vi "Generation word specific.vi"(11 "Template Path":path) -> ()   [LabVIEW 2020]
uses:
  <vilib>/Utility/NIReport.llb/Report Type.ctl
  <vilib>/addons/_office/_exclsub.llb/font.ctl
  <vilib>/Utility/NIReport.llb/Append Text Table to Report (wrap).vi
  <vilib>/addons/_office/word.llb/Word Edit Cell ([str]).vi
  <vilib>/Utility/NIReport.llb/NI_report.lvclass
  <vilib>/Utility/NIReport.llb/NI_ReportGenerationCore.lvlib
  <vilib>/Utility/NIReport.llb/Word/NI_Word.lvclass
  <vilib>/addons/_office/NI_ReportGenerationToolkit.lvlib
panel:
  in  "Data Set Name":string
  in  "error in (no error)":errorcluster
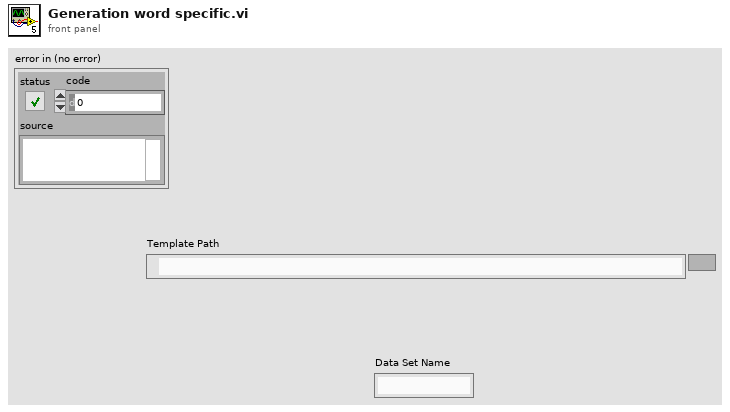
[diagram p1: front panel]
types:
  T1 = typedef "NI_ReportGenerationToolkit.lvlib/font.ctl" = cluster{"font name":string, "font size":dbl, "bold":u16, "italic":u16, "underline":u16, "strike through":u16, "font color":u32}
  T2 = typedef "NI_ReportGenerationCore.lvlib/Report Type.ctl" = enum16{"HTML", "Word", "Excel"}
  T3 = enum16{"maximized", "minimized", "normal", "no change"}
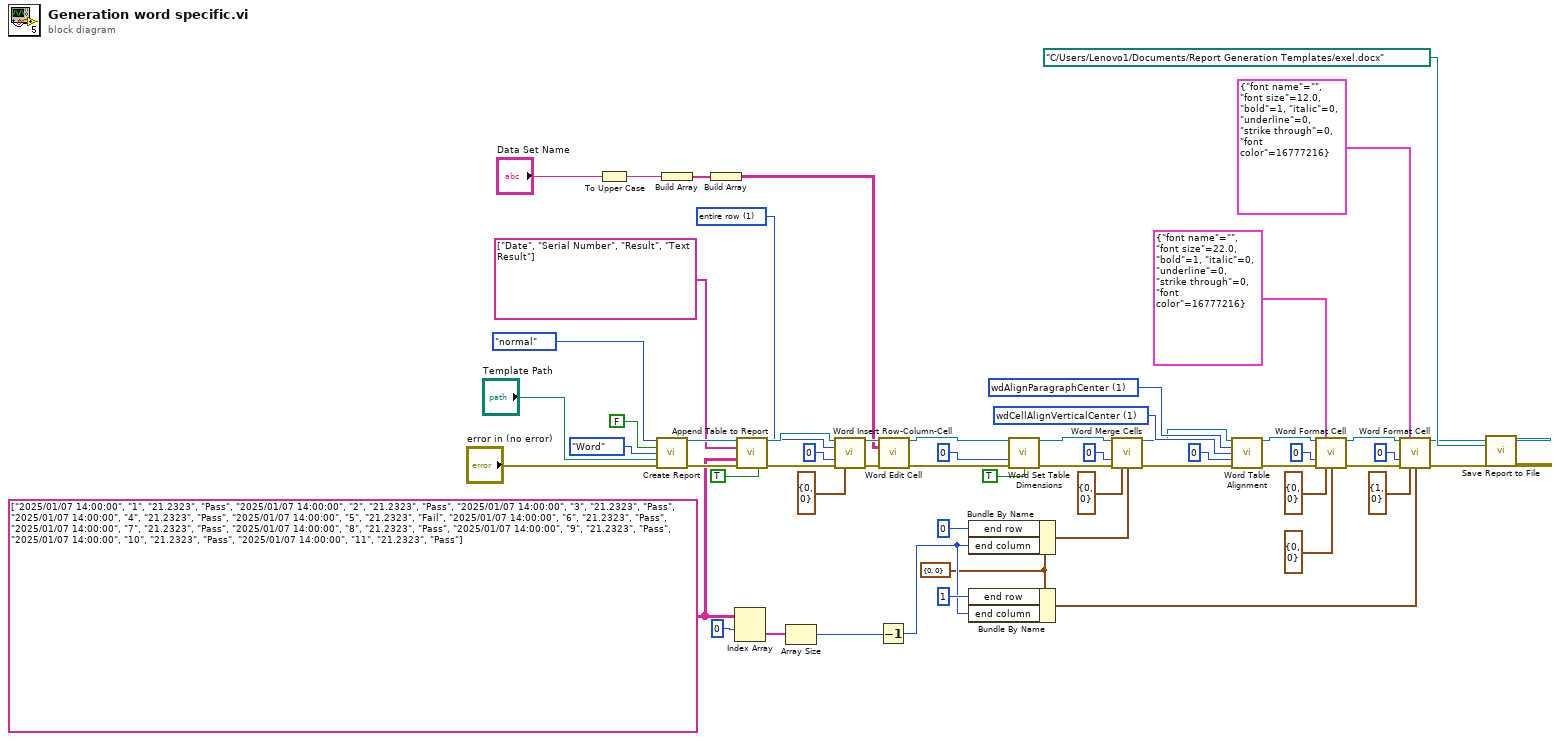
[diagram p0: block diagram]
diagram:
  w33 = u16 1 items=["shift cells right", "entire row", "entire column"] ("mode (entire column)")
  w1 = cluster{"end row":i32, "end column":i32} {"end row"=0, "end column"=0} ("end")
  w47 = 1 items=["wdCellAlignVerticalTop"=0, "wdCellAlignVerticalCenter"=1, "wdCellAlignVerticalBottom"=3] ("vertical alignment (top)")
  w48 = 1 items=["wdAlignParagraphLeft"=0, "wdAlignParagraphCenter"=1, "wdAlignParagraphRight"=2, "wdAlignParagraphJustify"=3, "wdAlignParagraphDistribute"=4, "wdAlignParagraphJustifyMed"=5, "wdAlignParagraphJustifyHi"=7, "wdAlignParagraphJustifyLow"=8] ("horizontal alignment (left)")
  w38 = string[][] [["2025/01/07 14:00:00", "1", "21.2323", "Pass"], ["2025/01/07 14:00:00", "2", "21.2323", "Pass"], ["2025/01/07 14:00:00", "3", "21.2323", "Pass"], ["2025/01/07 14:00:00", "4", "21.2323", "Pass"], ["2025/01/07 14:00:00", "5", "21.2323", "Fail"], ["2025/01/07 14:00:00", "6", "21.2323", "Pass"], ["2025/01/07 14:00:00", "7", "21.2323", "Pass"], ["2025/01/07 14:00:00", "8", "21.2323", "Pass"], ["2025/01/07 14:00:00", "9", "21.2323", "Pass"], ["2025/01/07 14:00:00", "10", "21.2323", "Pass"], ["2025/01/07 14:00:00", "11", "21.2323", "Pass"]] ("column headers")
  n1 = To Upper Case(1:"Data Set Name") -> (0:w7:string)
  n2 = call <vilib>:"Create Report.vi"("window state (normal)"=T3."normal", "display alerts? (F)"=FALSE, "report type"=Report_Type."Word", "template (empty)"="Template Path", "error in (no error)"="error in (no error)") -> ("report out"=w52:refnum<class "NI_report.lvclass">, "error out"=w51:errorcluster)  [unwired: 9 in]
  n3 = Build Array(w7) -> (w28:string[])
  n4 = Build Array(w28) -> (w27:string[][])
  n5 = Index Array(array=w38, index (row)=0) -> (element=w36:string[])  [unwired: 1 in]
  n6 = call-poly <vilib>:"Append Table to Report.vi"("report in"=w52, "column headers"=string[] ["Date", "Serial Number", "Result", "Text Result"], "text data"=w38, "error in (no error)"=w51, "show grid lines (YES)"=TRUE) -> ("report out"=w35:refnum<class "NI_report.lvclass">, "error out"=w34:errorcluster)  [unwired: 7 in, 2 out]
  n7 = Array Size(array=w36) -> (size(s)=w26:i32)
  n8 = call <vilib>:"Word Insert Row-Column-Cell.vi"("report in"=w35, "mode (entire column)"=w33, "table index (-1)"=i16 0, "error in (no error)"=w34, "start (0, 0)"=cluster{"row":i32, "column":i32} {"row"=0, "column"=0}) -> ("report out"=w30:refnum<class "NI_report.lvclass">, "error out"=w29:errorcluster)  [unwired: 9 in]
  n9 = Decrement(x=w26) -> (x-1=w3:i32)
  n10 = call-poly <vilib>:"Word Edit Cell.vi"("report in"=w30, "value"=w27, "error in (no error)"=w29) -> ("report out"=w25:refnum<class "NI_report.lvclass">, "error out"=w24:errorcluster)  [unwired: 11 in]
  n11 = Bundle By Name(cluster=w1, "end row"=0, "end column"=w3) -> (w40:cluster{"end row":i32, "end column":i32})
  n12 = Bundle By Name(cluster=w1, "end row"=1, "end column"=w3) -> (w2:cluster{"end row":i32, "end column":i32})
  n13 = call <vilib>:"Word Set Table Dimensions.vi"("report in"=w25, "table index (-1)"=i16 0, "error in (no error)"=w24, "fit to page width? (F)"=TRUE) -> ("report out"=w23:refnum<class "NI_report.lvclass">, "error out"=w22:errorcluster)  [unwired: 10 in]
  n14 = call <vilib>:"Word Merge Cells.vi"("report in"=w23, "table index (-1)"=i16 0, "error in (no error)"=w22, "start (0, 0)"=cluster{"start row":i32, "start column":i32} {"start row"=0, "start column"=0}, "end"=w40) -> ("report out"=w21:refnum<class "NI_report.lvclass">, "error out"=w20:errorcluster)  [unwired: 9 in]
  n15 = call <vilib>:"Word Table Alignment.vi"("report in"=w21, "horizontal alignment (left)"=w48, "vertical alignment (top)"=w47, "table index (-1)"=i16 0, "error in (no error)"=w20) -> ("report out"=w19:refnum<class "NI_report.lvclass">, "error out"=w18:errorcluster)  [unwired: 9 in]
  n16 = call <vilib>:"Word Format Cell.vi"("report in"=w19, "font"=T1 {"font name"="", "font size"=22.0, "bold"=1, "italic"=0, "underline"=0, "strike through"=0, "font color"=16777216}, "table index (-1)"=i16 0, "error in (no error)"=w18, "start (-1, -1)"=cluster{"start row":i32, "start column":i32} {"start row"=0, "start column"=0}, "end (-1, -1)"=cluster{"end row":i32, "end column":i32} {"end row"=0, "end column"=0}) -> ("report out"=w13:refnum<class "NI_report.lvclass">, "error out"=w12:errorcluster)  [unwired: 8 in]
  n17 = call <vilib>:"Word Format Cell.vi"("report in"=w13, "font"=T1 {"font name"="", "font size"=12.0, "bold"=1, "italic"=0, "underline"=0, "strike through"=0, "font color"=16777216}, "table index (-1)"=i16 0, "error in (no error)"=w12, "start (-1, -1)"=cluster{"start row":i32, "start column":i32} {"start row"=1, "start column"=0}, "end (-1, -1)"=w2) -> ("report out"=w11:refnum<class "NI_report.lvclass">, "error out"=w10:errorcluster)  [unwired: 8 in]
  n18 = call-dynamic "Save Report to File.vi"("report in"=w11, "report file path"=path "C:/Users/Lenovo1/Documents/Report Generation Templates/exel.docx", "error in (no error)"=w10) -> ()  [unwired: 11 in, 2 out]
